vi "Add Transition.vi"(7 "Input":string, 8 "error in (no error)":errorcluster, 9 "To State":string, 10 "From State":string, 11 "StateMachine in":refnum<class "StateMachine.lvclass">) -> (0 "error out":errorcluster, 3 "StateMachine out":refnum<class "StateMachine.lvclass">)   [LabVIEW 2019, in "State Machine.lvlib" / "StateMachine.lvclass"]
uses:
  StateMachine.lvclass
  StateMachine.lvclass/StateMachine.ctl
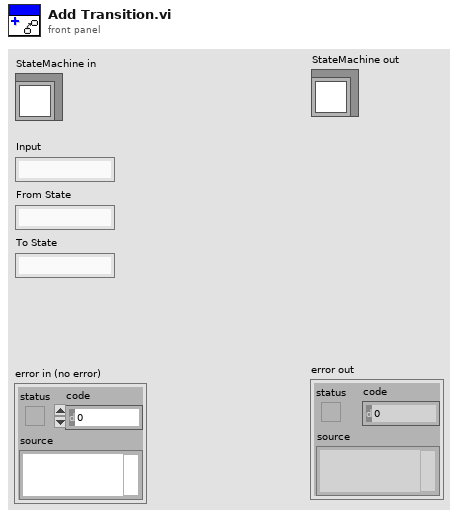
[diagram p1: front panel]
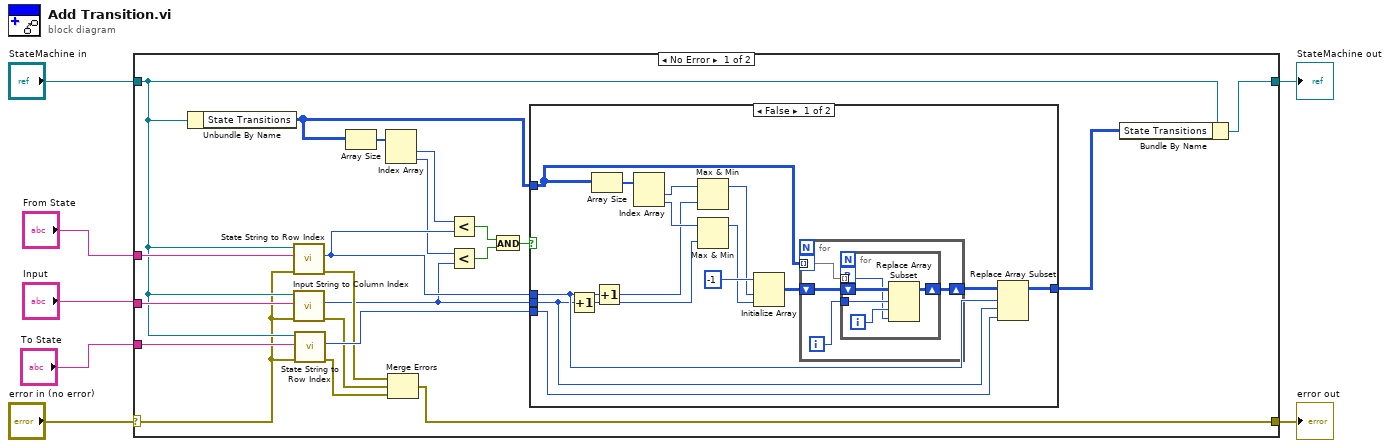
[diagram p0: block diagram]
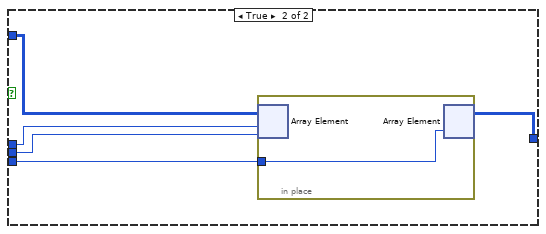
[diagram p2: hidden frame]
diagram:
  n1 = case shown="No Error" "error in (no error)" {
    selector: "error in (no error)" -> [w15 w60]
    tunnel: [w12 w60] -> w6
    tunnel: [w16 w59] -> w4
    tunnel: "StateMachine in" -> [w23 w59]
    tunnel: "From State" -> [w28 _]
    tunnel: "To State" -> [w27 _]
    tunnel: "Input" -> [w26 _]
    frame No Error {
      n2 = Unbundle By Name(w23) -> ("State Transitions"=w17:i32[][])
      n3 = call-dynamic "State String to Row Index.vi"("error in (no error)"=w15, "State String"=w28, "StateMachine in"=w23) -> ("error out"=w14:errorcluster, "Row Index"=w10:i32)  [unwired: 6 in, 1 out]
      n4 = call-dynamic "Input String to Column Index.vi"("error in (no error)"=w15, "Input String"=w26, "StateMachine in"=w23) -> ("error out"=w13:errorcluster, "Column Index"=w8:i32)  [unwired: 6 in, 1 out]
      n5 = call-dynamic "State String to Row Index.vi"("error in (no error)"=w15, "State String"=w27, "StateMachine in"=w23) -> ("error out"=w11:errorcluster, "Row Index"=w25:i32)  [unwired: 6 in, 1 out]
      n6 = Array Size(array=w17) -> (size(s)=w22:i32[])
      n7 = Index Array(array=w22) -> (element #1=w21:i32, element #2=w9:i32)  [unwired: 2 in]
      n8 = Merge Errors(w14, w13, w11) -> (w12:errorcluster)
      n9 = Less?(x=w21, y=w10) -> (x < y?=w20:bool)
      n10 = Less?(x=w9, y=w8) -> (x < y?=w19:bool)
      n11 = And(x=w20, y=w19) -> (x .and. y?=w18:bool)
      n12 = case shown="False" w18 {
        tunnel: w25 -> [w40 w54]
        tunnel: [w39 w53] -> w24
        tunnel: w17 -> [w36 w57]
        tunnel: w10 -> [w38 w56]
        tunnel: w8 -> [w37 w55]
        frame False {
          n13 = Increment(x=w37) -> (x+1=w31:i32)
          n14 = Array Size(array=w36) -> (size(s)=w35:i32[])
          n15 = Increment(x=w38) -> (x+1=w32:i32)
          n16 = Index Array(array=w35) -> (element #1=w34:i32, element #2=w33:i32)  [unwired: 2 in]
          n17 = Max & Min(x=w34, y=w32) -> (max(x,y)=w30:i32)  [unwired: 1 out]
          n18 = Max & Min(x=w33, y=w31) -> (max(x,y)=w29:i32)  [unwired: 1 out]
          n19 = Initialize Array(-1, w30, w29) -> (w42:i32[][])
          n20 = for {
            tunnel: w36 -> [w47] mode=indexing
            shift-right: [w44] -> w41
            shift-left: w42 -> [w46]
            workers-P: _ -> [_]
            i -> [w45]
            n21 = for {
              tunnel: w47 -> [w49] mode=indexing
              tunnel: w45 -> [w51]
              shift-right: [w48] -> w44
              shift-left: w46 -> [w52]
              workers-P: _ -> [_]
              i -> [w50]
              n22 = Replace Array Subset(array=w52, new element=w49, index (row)=w51, index (col)=w50) -> (w48:i32[][])
            }
          }
          n23 = Replace Array Subset(array=w41, new element=w40, index (row)=w38, index (col)=w37) -> (w39:i32[][])
        }
        frame True {
          n24 = in-place {
            in-place-border: w54 -> [w58]
            n25 = in-place-array #1(w57, w56, w55) -> ()  [unwired: 1 out]
            n26 = in-place-array #1(w58) -> (w53:i32[][])  [unwired: 2 out]
          }
        }
      }
      n27 = Bundle By Name(cluster=w23, "State Transitions"=w24) -> (w16:refnum<class "StateMachine.lvclass">)
    }
    frame Error {
    }
  }
  "error out" <- w6
  "StateMachine out" <- w4
